vi "create_list_items.vi"(8 "error in (no error)":errorcluster, 10 "FilePaths":path[](array[path])) -> (0 "error out":errorcluster)   [LabVIEW 2017]
doc: "creates a AnalysisListItem Object for each file that stores the necessary information to display the AnalysisList."
uses:
  Classes/AnalysisListItems/AnalysisListItems.lvclass
  global_variables.vi
  Classes/AnalysisList/AnalysisList.lvclass
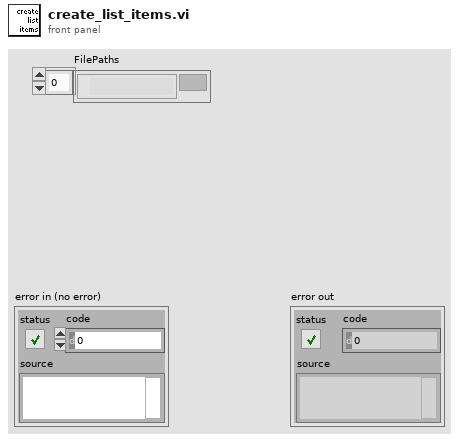
[diagram p1: front panel]
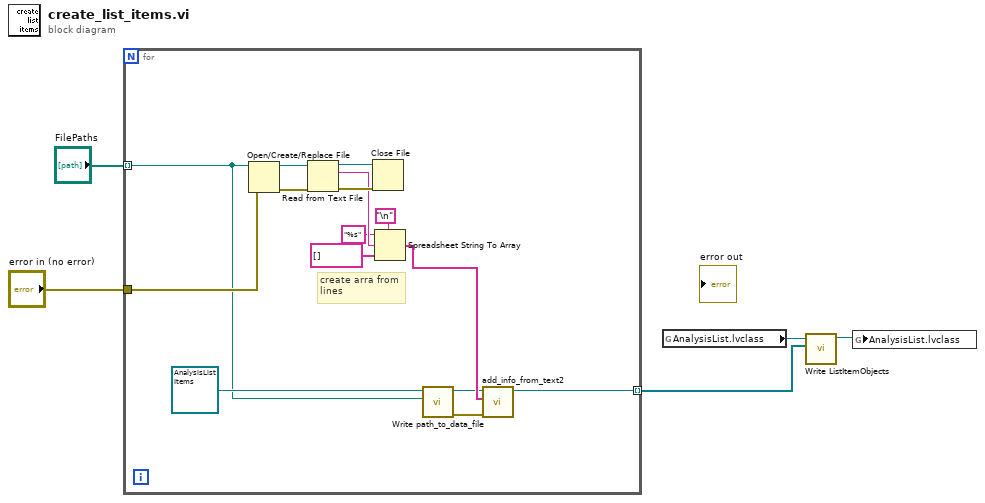
[diagram p0: block diagram]
diagram:
  n1 = for {
    tunnel: "FilePaths" -> [w6] mode=indexing
    tunnel: "error in (no error)" -> [w12]
    tunnel: [w10] -> w1 mode=indexing
    # "create arra from\nlines"
    n2 = Open/Create/Replace File(file path (use dialog)=w6, error in=w12) -> (refnum out=w20:refnum<file>, error out=w19:errorcluster)  [unwired: 4 in, 1 out]
    n3 = Read from Text File(file (use dialog)=w20, error in=w19) -> (refnum out=w18:refnum<file>, text=w15:string, error out=w17:errorcluster)  [unwired: 2 in, 1 out]
    n4 = Close File(refnum=w18, error in=w17) -> ()  [unwired: 2 out]
    n5 = Spreadsheet String To Array(delimiter (Tab)="\n", format string="%s", spreadsheet string=w15, array type (2D Dbl)=string[] []) -> (array=w11:string[])
    n6 = call-dynamic "Write path_to_data_file.vi"("path_to_data_file"=w6, "AnalysisListItems in"=refnum<class "AnalysisListItems.lvclass"> refnum ("AnalysisListItems.lvclass")) -> ("error out"=w8:errorcluster, "AnalysisListItems out"=w9:refnum<class "AnalysisListItems.lvclass">)  [unwired: 8 in]
    n7 = call-dynamic "add_info_from_text2.vi"("error in (no error)"=w8, "data array"=w11, "AnalysisListItems in"=w9) -> ("AnalysisListItems out"=w10:refnum<class "AnalysisListItems.lvclass">)  [unwired: 6 in, 2 out]
  }
  n8 = global read "global_variables.vi" "AnalysisList.lvclass"() -> (w3:refnum<class "AnalysisList.lvclass">)
  n9 = call-dynamic "Write ListItemObjects.vi"("AnalysisObjects"=w1, "AnalysisList in"=w3) -> ("AnalysisList out"=w2:refnum<class "AnalysisList.lvclass">)  [unwired: 8 in, 1 out]
  n10 = global write "global_variables.vi" "AnalysisList.lvclass"(w2) -> ()
